vi "Serialize Class.vi"(7 "Formatter":refnum<class "Formatter.lvclass">, 8 "error in":errorcluster, 10 "file path":path, 11 "Instrument in":refnum<class "Instrument.lvclass">) -> (0 "error out":errorcluster, 2 "JSON String":string, 3 "Instrument out":refnum<class "Instrument.lvclass">)   [LabVIEW 2012]
uses:
  <userlib>/Serialization/JSON Serializer/JSON Serializer.lvclass
  <userlib>/Serialization/Serializer/Serializer.lvclass
  Instrument.lvclass
  <userlib>/Serialization/Formatter/Formatter.lvclass
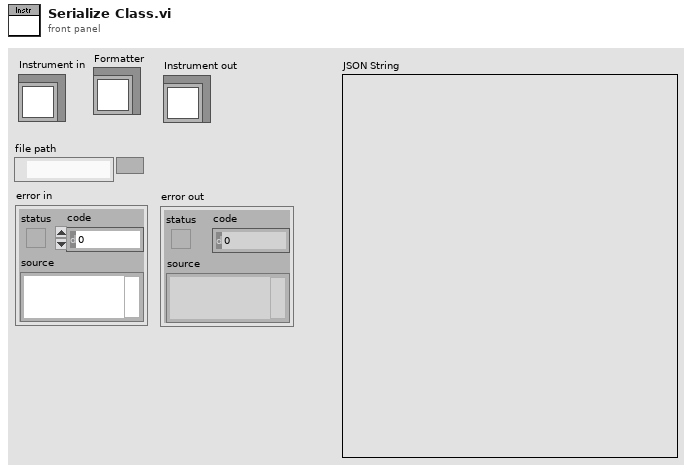
[diagram p1: front panel]
types:
  T1 = enum16{"open", "replace", "create", "open or create", "replace or create", "replace or create with confirmation"}
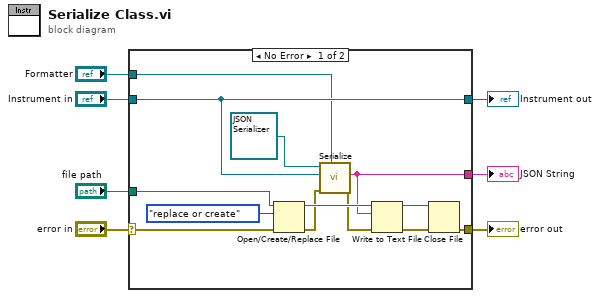
[diagram p0: block diagram]
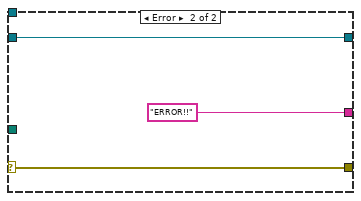
[diagram p2: hidden frame]
diagram:
  n1 = case shown="No Error" "error in" {
    selector: "error in" -> [w11 w23]
    tunnel: [w10 w23] -> w6
    tunnel: [w13 w22] -> w4
    tunnel: "Instrument in" -> [w13 w22]
    tunnel: [w12 "ERROR!!" ("String")] -> w3
    tunnel: "file path" -> [w9 _]
    tunnel: "Formatter" -> [w8 _]
    frame No Error {
      n2 = Open/Create/Replace File(file path (use dialog)=w9, error in=w11, operation (0:open)=T1."replace or create") -> (refnum out=w18:refnum<file>, error out=w15:errorcluster)  [unwired: 3 in, 1 out]
      n3 = call <userlib>:"Serialize.vi"("Formatter (defaults)"=w8, "error in (no error)"=w15, "Serializable"=w13, "Serializer"=refnum<class "JSON Serializer.lvclass"> refnum ("JSON Serializer.lvclass")) -> ("error out"=w14:errorcluster, "String"=w12:string)  [unwired: 5 in, 1 out]
      n4 = Write to Text File(file (use dialog)=w18, text=w12, error in=w14) -> (refnum out=w16:refnum<file>, error out=w17:errorcluster)  [unwired: 1 in, 1 out]
      n5 = Close File(refnum=w16, error in=w17) -> (error out=w10:errorcluster)  [unwired: 1 out]
    }
    frame Error {
    }
  }
  "error out" <- w6
  "Instrument out" <- w4
  "JSON String" <- w3
